vi "Database_simpletry_write.vi"() -> ()   [LabVIEW 2012]
uses:
  <vilib>/addons/database/Connection.llb/DB Tools Open Connec (Path).vi
  <vilib>/Analysis/1siggen.llb/Ramp Pattern by Samples.vi
  <vilib>/addons/database/NI_Database_API.lvlib
  <vilib>/Analysis/NI_AALBase.lvlib
panel:
  out "y":dbl[](graph)
  out "x":dbl[](graph)
  in  "stop":bool
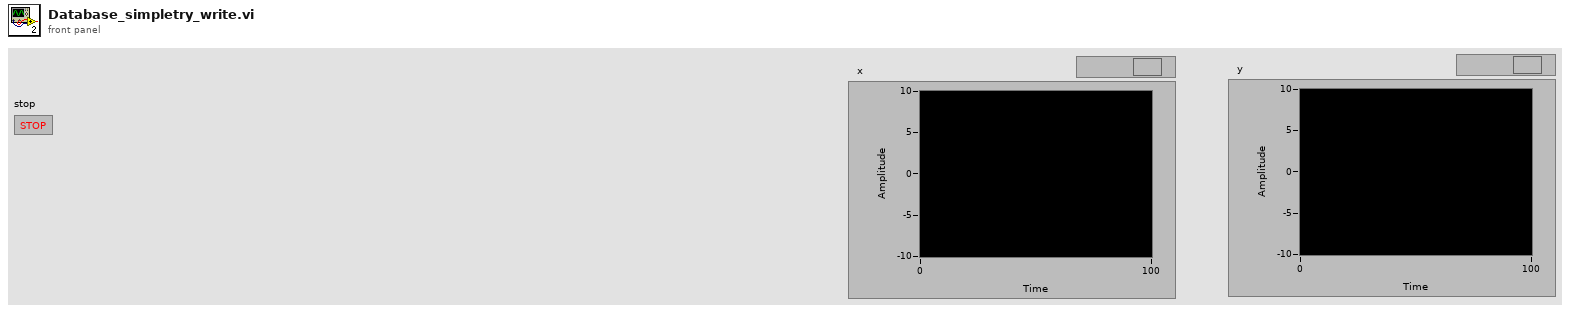
[diagram p1: front panel]
types:
  T1 = typedef "NI_Database_API.lvlib/Conn ObjectReference.ctl" = refnum<k1>
  T2 = cluster{"Ramp Pattern":dbl[], "Sinc Pattern":dbl[]}
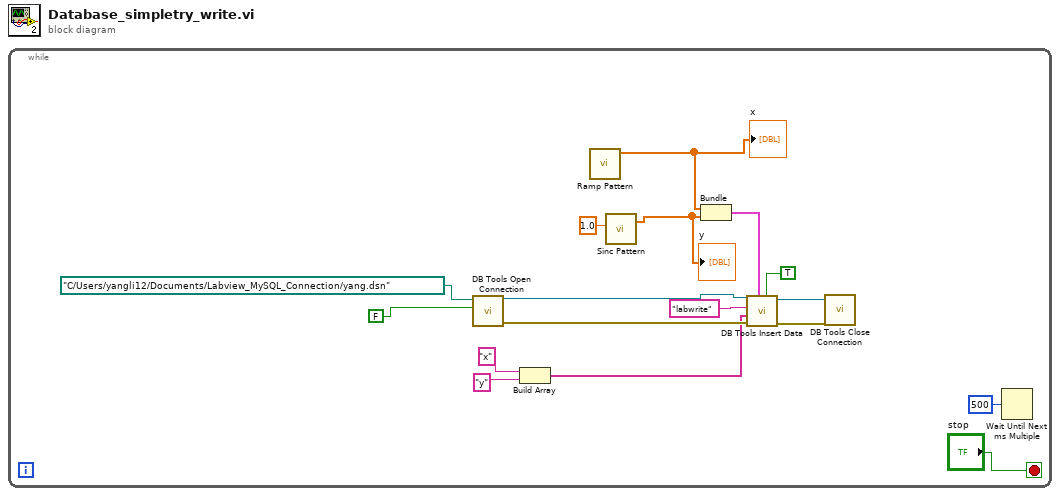
[diagram p0: block diagram]
diagram:
  n1 = while {
    stop <- "stop" stop-if-true
    n2 = call-poly <vilib>:"DB Tools Open Connection.vi"("prompt? (F)"=FALSE, "connection information"=path "C:/Users/yangli12/Documents/Labview_MySQL_Connection/yang.dsn") -> ("error out"=w11:errorcluster, "connection reference"=w12:T1)  [unwired: 6 in]
    n3 = Build Array("x" ("element"), "y" ("table")) -> (w9:string[])
    n4 = call-poly <vilib>:"Ramp Pattern.vi"() -> ("Ramp Pattern"=w1:dbl[])  [unwired: 10 in, 1 out]
    "x" <- w1
    n5 = call <vilib>:"Sinc Pattern.vi"("amplitude"=1.0) -> ("Sinc Pattern"=w2:dbl[])  [unwired: 3 in, 1 out]
    "y" <- w2
    n6 = Bundle("Ramp Pattern"=w1, "Sinc Pattern"=w2) -> (w4:T2)  [unwired: 1 in]
    n7 = call <vilib>:"DB Tools Insert Data.vi"("create table? (F)"=TRUE, "data"=w4, "error in (no error)"=w11, "columns"=w9, "table"="labwrite", "connection reference"=w12) -> ("error out"=w6:errorcluster, "connection reference out"=w7:T1)  [unwired: 4 in]
    n8 = call <vilib>:"DB Tools Close Connection.vi"("error in (no error)"=w6, "connection reference"=w7) -> ()  [unwired: 5 in, 1 out]
    n9 = Wait Until Next ms Multiple(millisecond multiple=u32 500) -> ()  [unwired: 1 out]
  }
